vi "Agilent E8257D module.vi"() -> ()   [LabVIEW 2020]
panel:
  out "error out":errorcluster
  in  "Power dbm":dbl
  in  "Frequency GHz":dbl
  in  "Output Enable":bool
  in  "error in (no error)":errorcluster
  in  "VISA resource name":refnum<visa-resource-name>
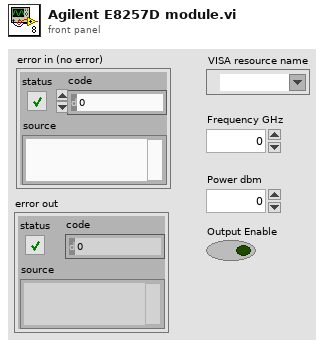
[diagram p1: front panel]
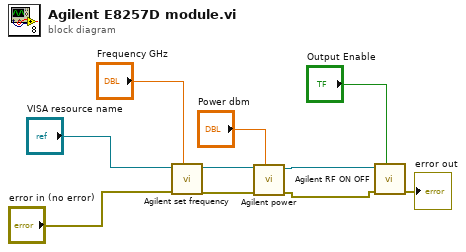
[diagram p0: block diagram]
diagram:
  n1 = call "Agilent set frequency.vi"("Frequency GHz"="Frequency GHz", "error in (no error)"="error in (no error)", "VISA resource name"="VISA resource name") -> ("error out"=w4:errorcluster, "VISA resource name out"=w8:refnum<visa-resource-name>)  [unwired: 7 in]
  n2 = call "Agilent power.vi"("Power dbm"="Power dbm", "error in (no error)"=w4, "VISA resource name"=w8) -> ("error out"=w5:errorcluster, "VISA resource name out"=w7:refnum<visa-resource-name>)  [unwired: 7 in]
  n3 = call "Agilent RF ON OFF.vi"("Output Enable"="Output Enable", "error in (no error)"=w5, "VISA resource name"=w7) -> ("error out"=→"error out":errorcluster)  [unwired: 7 in, 1 out]
